vi "robotIdEncoder.vi"(8 "error in (no error)":errorcluster, 9 "yellowteam":bool, 10 "id":u32, 11 "Communication in":refnum<class "Communication.lvclass">) -> (0 "error out":errorcluster, 1 "robotID Array":u8[](array[numeric]), 3 "Communication out":refnum<class "Communication.lvclass">)   [LabVIEW 2023, in "Communication.lvclass"]
uses:
  Communication.lvclass
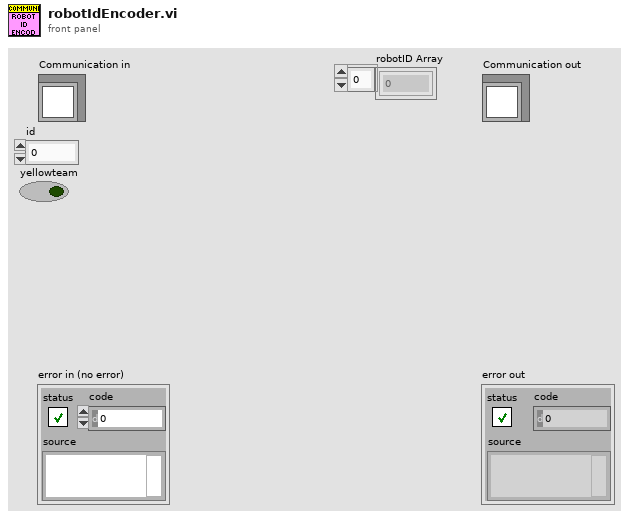
[diagram p1: front panel]
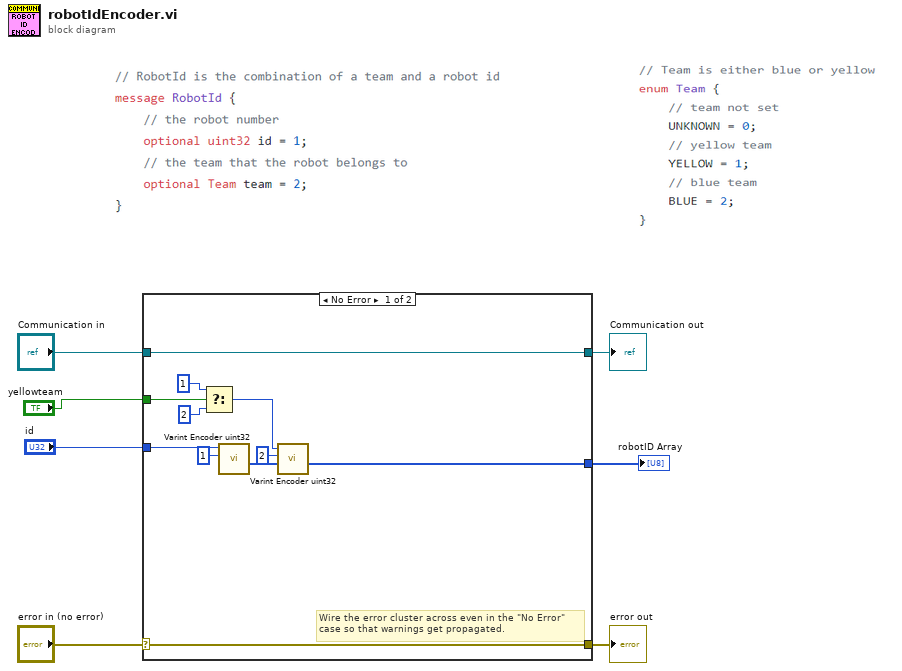
[diagram p0: block diagram]
diagram:
  n1 = case shown="No Error" "error in (no error)" {
    selector: "error in (no error)" -> [w17 w20]
    tunnel: [w17 w20] -> w6
    tunnel: [w18 w19] -> w4
    tunnel: "Communication in" -> [w18 w19]
    tunnel: "id" -> [w16 _]
    tunnel: [w12 _] -> w2
    tunnel: "yellowteam" -> [w11 _]
    frame No Error {
      # "Wire the error cluster across even in the \"No Error\"\ncase so that warnings get propagated."
      n2 = Select(t=u32 1 ("Key"), s=w11, f=u32 2 ("Key")) -> (s? t:f=w8:u32)
      n3 = call "Varint Encoder uint32.vi"("Key"=u32 1, "Value"=w16) -> ("Array"=w14:u8[])  [unwired: 9 in]
      n4 = call "Varint Encoder uint32.vi"("Array In"=w14, "Key"=u32 2, "Value"=w8) -> ("Array"=w12:u8[])  [unwired: 8 in]
    }
    frame Error {
    }
  }
  "error out" <- w6
  "Communication out" <- w4
  "robotID Array" <- w2
